vi "ClientSDO_connect.vi"(8 "error in (no error)":errorcluster, 9 "node_id":u8, 10 "bitrate":i32, 11 "port":i32) -> (0 "error out":errorcluster, 2 "canHardwareConnect":i32(ring) items=["CANOPEN_OK"=0, "CANOPEN_ERROR"=-255, "CANOPEN_ERROR_ASYNC_TRANSFER_ENABLED"=-114, "CANOPEN_ASYNC_TRANSFER"=-113, "CANOPEN_ERROR_NOT_EDS_DCF_CONFIGURED"=-112, "CANOPEN_ERROR_FILE_NOT_FOUND"=-111, "CANOPEN_ERROR_NOT_IMPLEMENTED"=-110, "CANOPEN_ERROR_NO_MESSAGE"=-109, "CANOPEN_UNSUPPORTED_BITRATE"=-108, "CANOPEN_OUT_OF_CAN_INTERFACES"=-107, "CANOPEN_ERROR_DRIVER"=-106, "CANOPEN_ERROR_HW_UNDEFINED"=-105, "CANOPEN_ERROR_HW_NOT_CONNECTED"=-104, "CANOPEN_ERROR_HW_CONNECTED"=-103, "CANOPEN_ERROR_CAN_LAYER_OVRFLOW"=-102, "CANOPEN_ERROR_CAN_LAYER"=-101, "CANOPEN_CAN_LAYER_FAILED"=-100, "CANOPEN_NODE_ID_OUT_OF_RANGE"=-15, "CANOPEN_INTERNAL_STATE_ERROR"=-14, "CANOPEN_CMD_SPEC_UNKNOWN_OR_INVALLD"=-13, "CANOPEN_ERR_DEFINED_BY_APPL"=-12, "CANOPEN_OUT_OF_MEM"=-11, "CANOPEN_REMOTE_NODE_ABORT"=-10, "CANOPEN_APP_BUF_OUT_OF_RANGE"=-9, "CANOPEN_OBJECT_MISSMATCH"=-8, "CANOPEN_BUFFER_TOO_SMALL"=-7, "CANOPEN_TOGGLE"=-6, "CANOPEN_MSG_NOT_PROCESSED"=-5, "CANOPEN_TIMEOUT"=-4, "CANOPEN_UNEXPECTED_CCS"=-3, "CANOPEN_UNEXPECTED_SCS"=-2, "CANOPEN_ARG_ERROR"=-1], 3 "ClientSDO Ref out":refnum<k24>)   [LabVIEW 2015, in "CANOpen.lvlib"]
doc: "connect to client CANOpen device for writting/reading data using SDO protocol."
uses:
  CANOpen.lvlib
  \\Mac\Home/Desktop/imt_test_app 28-06-2012/canopenlib_cli.dll
  canopenlib_cli.dll
panel:
  out "error out 2":errorcluster
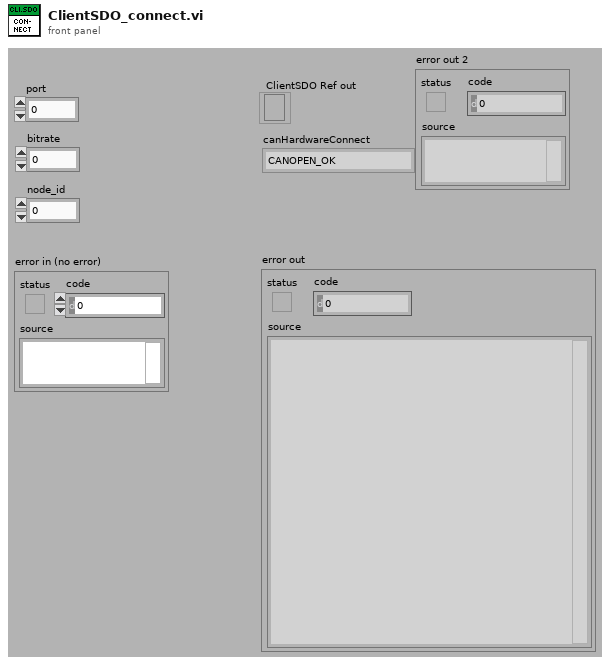
[diagram p1: front panel]
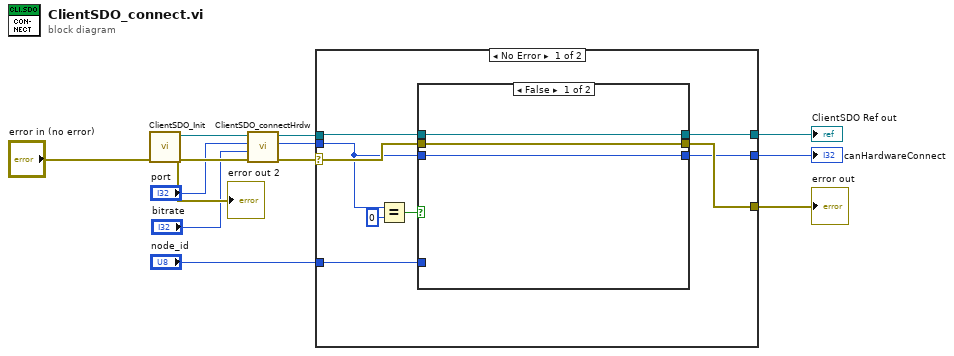
[diagram p0: block diagram]
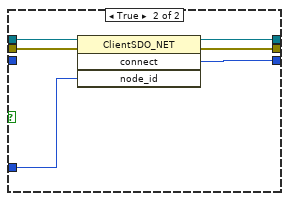
[diagram p2: hidden frame]
diagram:
  n1 = call "ClientSDO_Init.vi"("error in (no error)"="error in (no error)") -> ("error out"=w11:errorcluster, "ClientSDO Ref out"=w12:refnum<k24>)  [unwired: 9 in]
  "error out 2" <- w11
  n2 = call "ClientSDO_connectHrdw.vi"("error in (no error)"=w11, "bitrate"="bitrate", "port"="port", "ClientSDO Ref in"=w12) -> ("error out"=w8:errorcluster, "canHardwareConnect"=w6:i32, "ClientSDO Ref out"=w7:refnum<k24>)  [unwired: 5 in]
  n3 = case shown="No Error" w8 {
    selector: w8 -> [w18 w32]
    tunnel: w7 -> [w21 w33]
    tunnel: w6 -> [w13 w31]
    tunnel: "node_id" -> [w17 _]
    tunnel: [w16 w33] -> w4
    tunnel: [w15 w32] -> w1
    tunnel: [w14 w31] -> w3
    frame No Error {
      n4 = Equal?(x=w13, y=0) -> (x = y?=w19:bool)
      n5 = case shown="False" w19 {
        tunnel: w21 -> [w24 w30]
        tunnel: w18 -> [w23 w29]
        tunnel: w17 -> [_ w28]
        tunnel: [w24 w27] -> w16
        tunnel: [w23 w26] -> w15
        tunnel: [w22 w25] -> w14
        tunnel: w13 -> [w22 _]
        frame False {
        }
        frame True {
          n6 = invoke class="ClientSDO_NET" method="connect"(reference=w30, error in=w29, "node_id"=w28) -> (reference out=w27:refnum<k24>, error out=w26:errorcluster, "connect"=w25:i32)  [unwired: 1 in, 1 out]
        }
      }
    }
    frame Error {
    }
  }
  "ClientSDO Ref out" <- w4
  "error out" <- w1
  "canHardwareConnect" <- w3
